vi "Moment about Mean.vi"(2 "order":i32=2, 3 "X":dbl[](array[numeric]) format="%0.2f") -> (0 "error":i32, 1 "moment":dbl format="%0.2f")   [LabVIEW 2017, in "NI_AALPro.lvlib"]
doc: "Computes the moment about the mean of the input sequence <B>X</B> using the specified <B>order</B>, m."
uses:
  <vilib>/Analysis/NI_AALPro.lvlib
  <resource>/lvanlys.dll
panel:
  # "Moment about Mean"
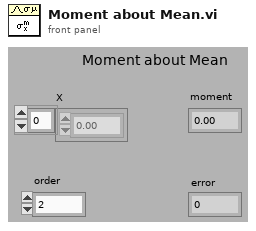
[diagram p1: front panel]
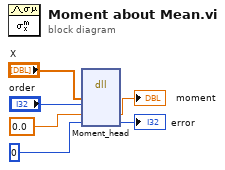
[diagram p0: block diagram]
diagram:
  n1 = dll-call lib="e:/builds/penguin/labview/branches/2017/dev/dist/resource/lvanlys.*" fn="Moment_head"("X"="X", "order"="order", "moment"=0.0, "error"=0) -> ("moment"=→"moment":dbl, "error"=→"error":i32)  [unwired: 6 in, 2 out]
